vi "运维调试_总磷总氮.vi"() -> ()   [LabVIEW 2016, in "斯坦道氨氮.lvlib"]
uses:
  <vilib>/Utility/miscctls.llb/LVPointTypeDef.ctl
  <vilib>/Plasmionique/MB Master/MB_Master/MB_Master.lvclass
  <vilib>/Utility/config.llb/NI_LVConfig.lvlib
  <vilib>/ptbypt/NI_PtbyPt.lvlib
panel:
  out "权限等级":enum16{"一级权限", "二级权限", "三级权限", "超级权限"}(ring)
  out "试剂余量显示":sgl[][](graph)
  in  "仪器校准":bool
  in  "参数查询":bool
  out "简易步骤名称":string
  in  "温度曲线":bool
  in  "试剂余量":bool
  in  "灯值调整":bool
  in  "启动参数设置":bool
  out "固件版本号":string
  in  "定时设置":cluster{"启动":bool, "控制命令":T1, "测量参数":T2}(xcontrol)
  out "模块版本号":string
  out "注射器温度":sgl
  out "消解温度":sgl
  out "ADC":sgl
  out "F3":sgl format="%#.6f"
  out "F2":sgl format="%#.6f"
  out "F1":sgl format="%#.6f"
  out "F0":sgl format="%#.6f"
  out "运行状态":T3 {"数据时间:" format="%<%y/%m/%d %H:%M:%S>T"; "仪器时间:" format="%<%y/%m/%d %H:%M:%S>T"}
  in  "单选按钮":T4(radio)=enum."总氮"
  out "布尔":bool
  in  "流程固件":bool
  out "字符串 2":string
  in  "数组":string[](array[string])
  in  "返回":bool
  in  "参数设置":bool
  out "集成报警信息":string
  in  "停止":bool
  in  "手动启动":bool
  in  "调试":bool
  out "多列列表框":i32(listbox)
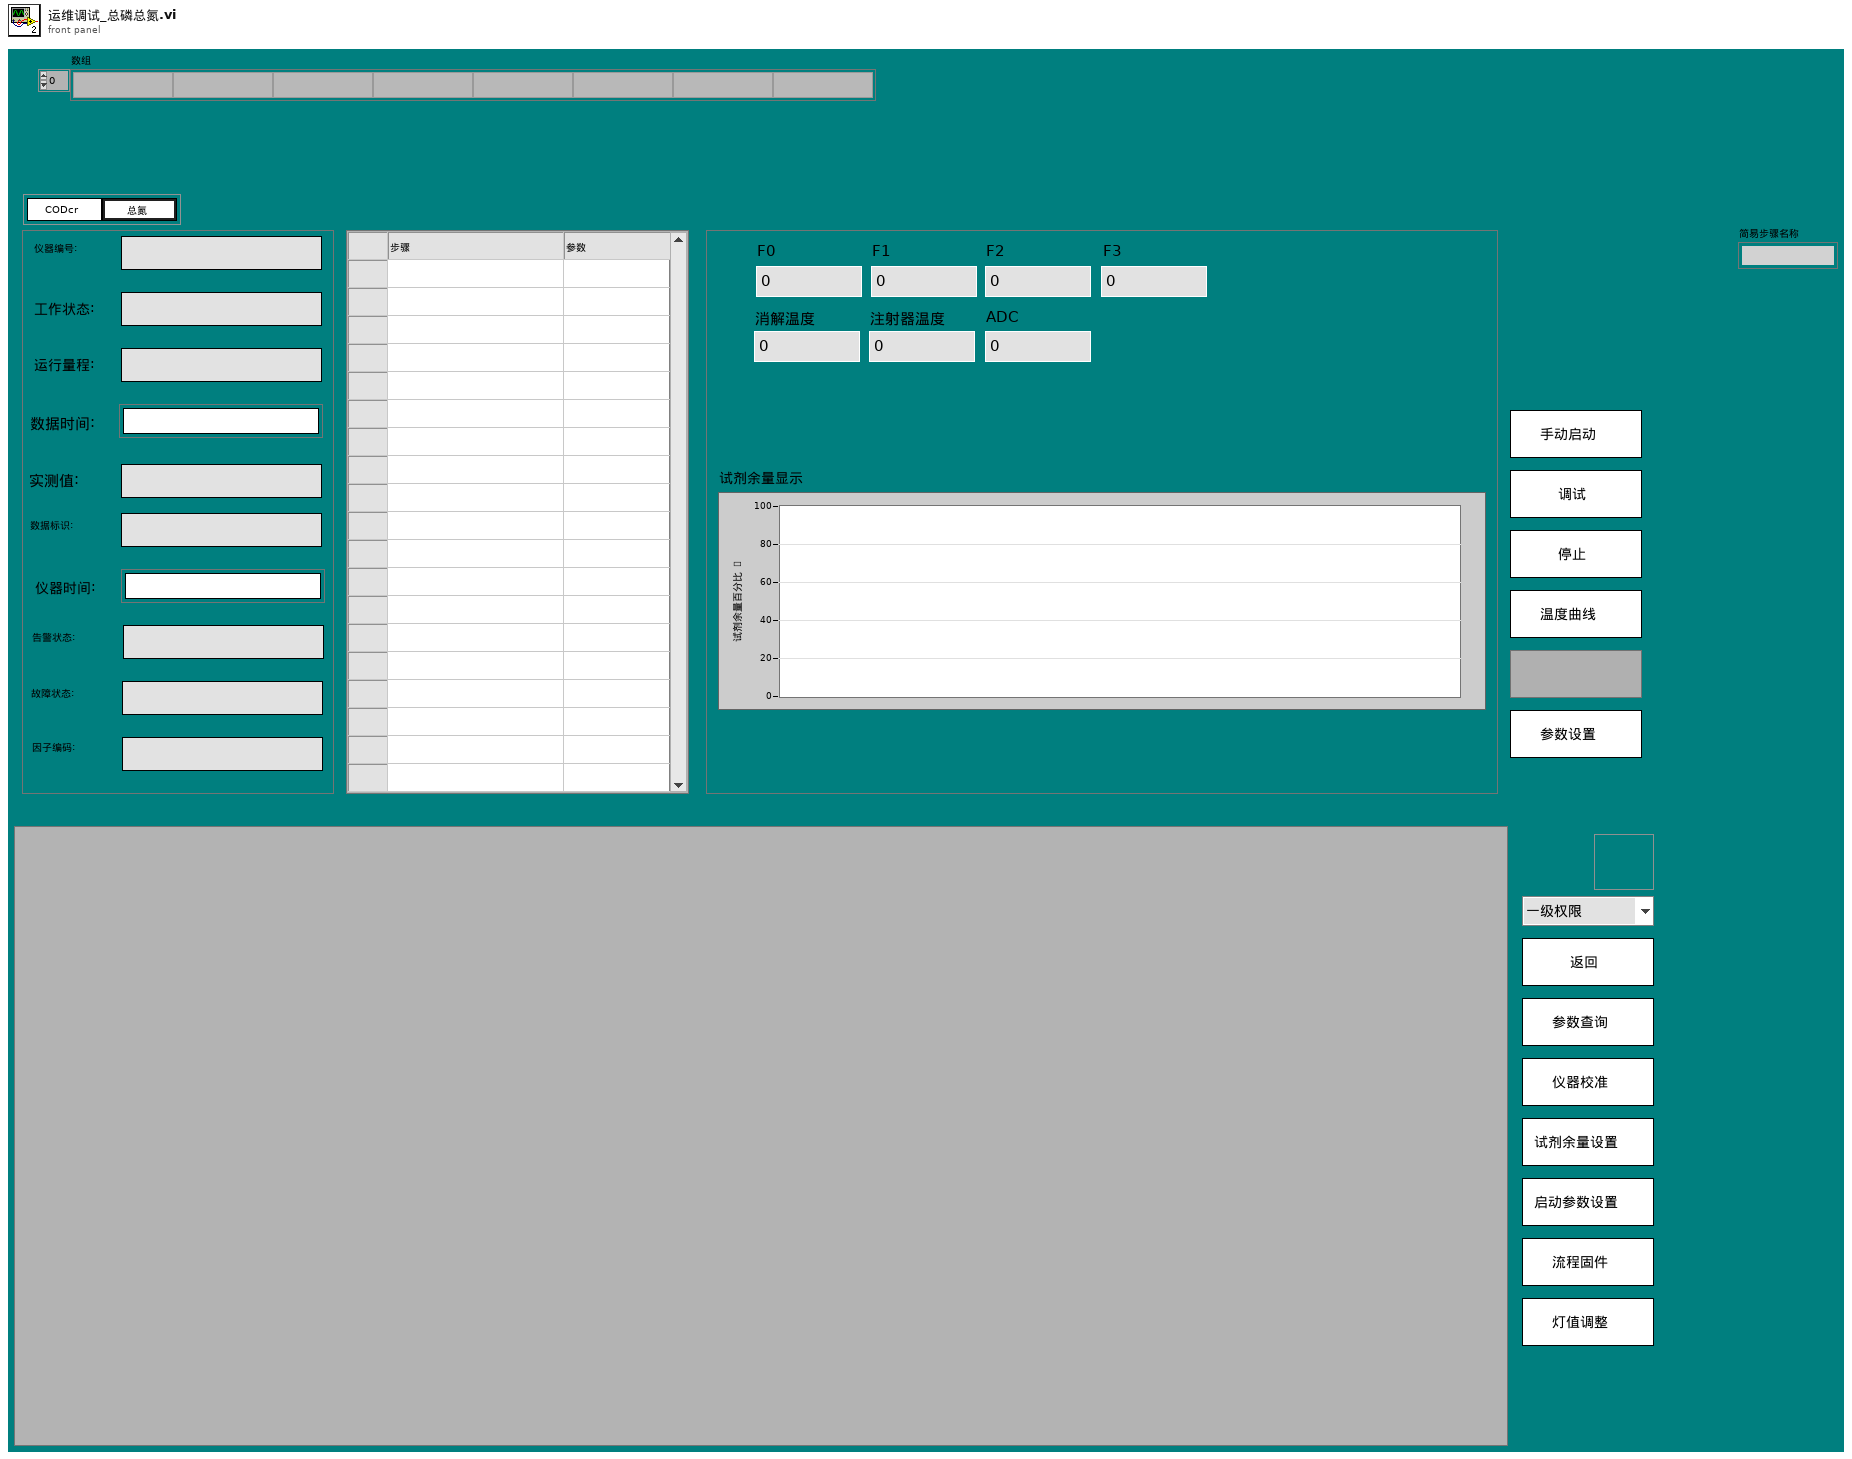
[diagram p1: front panel]
types:
  T1 = typedef "定时设置.xctl/国标控制命令.ctl" = enum16{"启动测量", "标样核查", "零点核查", "跨度核查", "空白测试", "平行样测试", "加标回收", "空白校准", "标样校准", "初始化（清洗）", "停止测试", "仪器重启", "校时", "模式设置", "测量间隔设置"}
  T2 = typedef "定时设置.xctl/测量参数.ctl" = u16
  T3 = cluster{"仪器编号:":string, "工作状态:":string, "运行量程: ":string, "数据时间:":timestamp, "实测值:":string, "数据标识: ":string, "仪器时间:":timestamp, "告警状态: ":string, "故障状态:  ":string, "因子编码:":string}
  T4 = enum32{"COD", "氨氮", "总氮", "总磷", "磷酸盐", "硝氮", "亚硝氮", "硅酸盐", "硫化物"}
  T5 = cluster{"时间源选择":enum16{"系统时间源", "仪器时间源"}, "外部时间源":timestamp}
  T6 = cluster{"系统时间":timestamp, "工作状态":u16, "测量模式":enum16{"待机", "连续模式", "周期模式", "定点模式", "受控模式", "手动模式"}, "告警代码":u16, "故障代码":u16, "日志代码":u16, "软件版本":u16, "F0":sgl, "F1":sgl, "F2":sgl, "F3":sgl, "T":sgl, "H":sgl, "id":u16, "flowid":u16, "量程":u16, "总磷控温温度1":sgl, "营养盐控温温度2":sgl, "ADC":sgl}
  T7 = enum32{"Bad", "Idle", "Run top level", "Running"}
  T8 = cluster{"Major":u16, "Minor":u16, "Fix":u16, "Build":u16}
  T9 = typedef "LVPointTypeDef.ctl" = cluster{"Horizontal":i16, "Vertical":i16}
  T10 = cluster{"因子编码":u32, "单位":u16, "标样参考值":sgl, "水样数据时间":timestamp, "水样实测值":sgl, "水样数据标识":string, "标样数据时间":timestamp, "标样实测值":sgl, "标样数据标识":string, "空白数据时间":timestamp, "空白实测值":sgl, "空白数据标识":string, "零点核查数据时间":timestamp, "零点核查实测值":sgl, "零点核查数据标识":string, "跨度核查数据时间":timestamp, "跨度核查实测值":sgl, "跨度核查数据标识":string, "加标回收数据时间":timestamp, "加标回收实测值":sgl, "加标回收数据标识":string, "平行样数据时间":timestamp, "平行样实测值":sgl, "平行样数据标识":string, "F0":sgl, "F1":sgl, "F2":sgl, "F3":sgl, "F4":sgl, "F5":sgl, "F6":sgl, "F7":sgl, "温度":sgl, "湿度":sgl, "X值":sgl, "fidrange":u16}[]
  T11 = cluster{"因子编码":u32, "单位":u16, "标样参考值":sgl, "水样数据时间":timestamp, "水样实测值":sgl, "水样数据标识":string, "标样数据时间":timestamp, "标样实测值":sgl, "标样数据标识":string, "空白数据时间":timestamp, "空白实测值":sgl, "空白数据标识":string, "零点核查数据时间":timestamp, "零点核查实测值":sgl, "零点核查数据标识":string, "跨度核查数据时间":timestamp, "跨度核查实测值":sgl, "跨度核查数据标识":string, "加标回收数据时间":timestamp, "加标回收实测值":sgl, "加标回收数据标识":string, "平行样数据时间":timestamp, "平行样实测值":sgl, "平行样数据标识":string, "F0":sgl, "F1":sgl, "F2":sgl, "F3":sgl, "F4":sgl, "F5":sgl, "F6":sgl, "F7":sgl, "温度":sgl, "湿度":sgl, "X值":sgl, "fidrange":u16}
  T12 = cluster{"时间标识":timestamp, "设备":string, "日志信息":string, "备注":string}
  T13 = cluster{"参数":string, "报警内容":string, "报警分析":string}
  T14 = typedef "NI_LVConfig.lvlib/Config Data RefNum.ctl" = refnum<k1>
  T15 = cluster{"时间标识":timestamp, "设备":string, "日志信息":string, "流程参数":string}
  T16 = typedef "LVRowAndColumnUnsignedTypeDef.ctl" = cluster{"Row":u32, "Column":u32}
  T17 = enum16{"空闲", "水样测试", "标样核查", "零点核查", "跨度核查", "空白测试", "平行样测试", "加标回收", "空白校准", "标样校准", "初始化（清洗）"}
  T18 = cluster{"站号":u16, "量程切换":enum32{"H", "L", "AUTO"}, "控制命令":enum16{"启动测量", "标样核查", "零点核查", "跨度核查", "空白测试", "平行样测试", "加标回收", "空白校准", "标样校准", "初始化（清洗）", "停止测试", "仪器重启", "校时", "模式设置", "测量间隔设置"}, "模式设置":enum16{"待机", "连续模式", "周期模式", "定点模式", "受控模式", "手动模式"}, "测量间隔":u16}
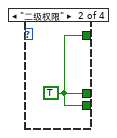
[diagram p9: hidden frame]
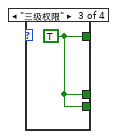
[diagram p10: hidden frame]
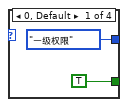
[diagram p11: hidden frame]
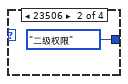
[diagram p12: hidden frame]
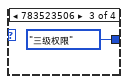
[diagram p13: hidden frame]
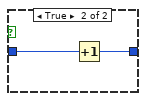
[diagram p15: hidden frame]
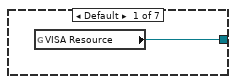
[diagram p17: hidden frame]
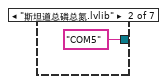
[diagram p18: hidden frame]
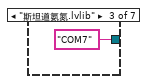
[diagram p19: hidden frame]
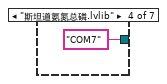
[diagram p20: hidden frame]
diagram:
  n1 = while {
    stop <- FALSE stop-if-true
    n2 = vi-ref "测量流程.vi"() -> (w39:refnum<vi>)
    n3 = global read "VAR总磷总氮全局变量.vi" "状态告警区"() -> (w36:T6)
    n4 = Wait (ms)(milliseconds to wait=u32 500 ("等待时间（毫秒）")) -> ()  [unwired: 1 out]
    n5 = Unbundle By Name("定时设置") -> ("启动"=w33:bool, "控制命令"=w32:T1)
    n6 = property class="VI"(reference=w39) -> ("Exec.State"=w38:T7, "Name"=w37:string)  [unwired: 1 in, 2 out]
    n7 = Unbundle By Name(w36) -> ("工作状态"=w35:u16, "系统时间"=w30:timestamp)
    n8 = case shown="真" w33 {
      tunnel: w37 -> [_ w46]
      tunnel: w32 -> [_ w45]
      tunnel: w38 -> [_ w44]
      frame False {
      }
      frame True {
        n9 = case shown="\"Idle\"" w44 {
          tunnel: w46 -> [_ w50]
          tunnel: w45 -> [_ w47]
          frame "Bad", Default {
          }
          frame "Idle" {
            n10 = Open VI Reference(type specifier VI Refnum (for type only)=refnum<vi> refnum, vi path=w50, options=128 ("选项")) -> (vi reference=w51:refnum<vi>, error out=w52:errorcluster)  [unwired: 3 in]
            n11 = call-by-ref "开始异步调用"(reference=w51, error in=w52, "控制命令"=w47) -> (reference out=w53:refnum<vi>, error out=w54:errorcluster)  [unwired: 11 in]
            n12 = Close Reference(reference=w53, error in (no error)=w54) -> ()  [unwired: 1 out]
          }
        }
      }
    }
    n13 = case shown="0" w35 {
      tunnel: [FALSE TRUE] -> w28
      frame 0 {
      }
      frame 1, Default {
      }
    }
    n14 = Bundle By Name(cluster=T5 {"时间源选择"=enum."仪器时间源", "外部时间源"=timestamp(0 s since 1904-01-01)} ("时间源"), "外部时间源"=w30) -> (w29:T5)
    n15 = property on="定时设置" class="定时设置 (严格)"("仪器状态"=w28, "时间源"=w29) -> ()  [unwired: 2 in, 2 out]
  }
  n16 = flat-sequence {
    tunnel: [w56] -> w16
    tunnel: [w55] -> w14
    tunnel: w16 -> [w67]
    tunnel: [w67] -> w15
    tunnel: w14 -> [w72]
    tunnel: [w72] -> w13
    tunnel: w15 -> [w98]
    tunnel: [w98] -> w17
    tunnel: w13 -> [_]
    tunnel: w17 -> [w101]
    tunnel: [w164] -> w18
    frame #0 {
      n17 = control-ref of="本VI"() -> (w66:refnum<vi>)
      n18 = property class="VI"(reference=w66) -> ("Library.Version"=w65:T8)  [unwired: 1 in, 2 out]
      n19 = Unbundle By Name(w65) -> ("Major"=w63:u16, "Minor"=w62:u16, "Fix"=w61:u16, "Build"=w60:u16)
      n20 = control-ref of="本VI"() -> (w57:refnum<vi>)
      n21 = Format Into String(format string="模块版本号：%d.%d.%d.%d" ("格式字符串"), w63, w62, w61, w60) -> (resulting string=→"模块版本号":string)  [unwired: 2 in, 1 out]
      n22 = property class="VI"(reference=w57) -> ("Library"=w58:refnum<vi>)  [unwired: 1 in, 2 out]
      n23 = property class="Library"(reference=w58) -> ("LocalName"=w56:string)  [unwired: 1 in, 2 out]
      n24 = property on="定时设置" class="定时设置 (严格)"("引用参数"=w56) -> ()  [unwired: 2 in, 2 out]
      n25 = call "配置读取.vi"() -> ("error out"=w55:errorcluster)  [unwired: 11 in]
    }
    frame #1 {
      n26 = global read "总磷总氮断电保存全局变量.vi" "IP"() -> (w71:string)
      n27 = global read "总磷总氮断电保存全局变量.vi" "VISA Resource"() -> (w68:refnum<visa-resource-name>)
      n28 = Empty String/Path?(string/path=w71) -> (empty?=w70:bool)
      n29 = case shown="真" w70 {
        tunnel: w67 -> [_ w83]
        frame False {
        }
        frame True {
          n30 = case shown="\"斯坦道CODcr.lvlib\"" w83 {
            tunnel: [w84 "192.168.1.203" ("IP") "192.168.1.202" ("IP") "192.168.1.202" ("IP") "192.168.1.203" ("IP") "192.168.1.204" ("IP") "192.168.1.205" ("IP")] -> w82
            frame Default {
              n31 = global read "总磷总氮断电保存全局变量.vi" "IP"() -> (w84:string)
            }
            frame "斯坦道总磷总氮.lvlib" {
            }
            frame "斯坦道氨氮.lvlib" {
            }
            frame "斯坦道氨氮总磷.lvlib" {
            }
            frame "斯坦道总磷.lvlib" {
            }
            frame "斯坦道总氮.lvlib" {
            }
            frame "斯坦道CODcr.lvlib" {
            }
          }
          n32 = global write "总磷总氮断电保存全局变量.vi" "IP"(w82) -> ()
        }
      }
      n33 = Empty String/Path?(string/path=w68) -> (empty?=w69:bool)
      n34 = case shown="真" w69 {
        tunnel: w67 -> [_ w74]
        frame False {
        }
        frame True {
          n35 = case shown="\"斯坦道CODcr.lvlib\"" w74 {
            tunnel: [w75 "COM5" ("IP") "COM7" ("IP") "COM7" ("IP") "COM5" ("IP") "COM10" ("IP") "COM9" ("IP")] -> w73
            frame Default {
              n36 = global read "总磷总氮断电保存全局变量.vi" "VISA Resource"() -> (w75:refnum<visa-resource-name>)
            }
            frame "斯坦道总磷总氮.lvlib" {
            }
            frame "斯坦道氨氮.lvlib" {
            }
            frame "斯坦道氨氮总磷.lvlib" {
            }
            frame "斯坦道总磷.lvlib" {
            }
            frame "斯坦道总氮.lvlib" {
            }
            frame "斯坦道CODcr.lvlib" {
            }
          }
          n37 = global write "总磷总氮断电保存全局变量.vi" "VISA Resource"(w73) -> ()
        }
      }
    }
    frame #2 {
      n38 = global read "总磷总氮断电保存全局变量.vi" "MB通信方式选择"() -> (w94:enum16{"串口", "TCP"})
      n39 = global read "总磷总氮断电保存全局变量.vi" "VISA Resource"() -> (w93:refnum<visa-resource-name>)
      n40 = global read "总磷总氮断电保存全局变量.vi" "PORT"() -> (w96:string)
      n41 = Decimal String To Number(string=w96) -> (number=w95:i32)  [unwired: 2 in, 1 out]
      n42 = global read "总磷总氮断电保存全局变量.vi" "IP"() -> (w97:string)
      n43 = call "获取启动参数.vi"("MB通信方式选择"=w94, "Port (502)"=w95, "IP Address"=w97, "VISA Resource"=w93) -> ("error out"=w92:errorcluster, "数组"=w91:cluster{"String":string, "Value":u16}[])  [unwired: 6 in]
      n44 = case shown="无错误" w92 {
        tunnel: w91 -> [w99 _]
        frame No Error {
          n45 = flat-sequence {
            tunnel: w99 -> [w100]
            frame #0 {
              n46 = global write "总磷总氮断电保存全局变量.vi" "启动队列名称"(w100) -> ()
            }
            frame #1 {
              n47 = call "配置写入.vi"() -> ()  [unwired: 11 in, 1 out]
            }
          }
        }
        frame Error {
        }
      }
    }
    frame #3 {
      n48 = global read "总磷总氮断电保存全局变量.vi" "启动队列名称"() -> (w103:cluster{"String":string, "Value":u16}[])
      n49 = Empty Array?(array=w103) -> (empty?=w102:bool)
      n50 = case shown="真" w102 {
        tunnel: w101 -> [_ w104]
        frame False {
        }
        frame True {
          n51 = case shown="\"斯坦道CODcr.lvlib\"" w104 {
            frame Default {
            }
            frame "斯坦道总磷总氮.lvlib" {
              n52 = global write "总磷总氮断电保存全局变量.vi" "启动队列名称"(cluster{"String":string, "Value":u16}[] [{"String"="总氮", "Value"=2}, {"String"="总磷", "Value"=1}] ("启动队列名称")) -> ()
            }
            frame "斯坦道氨氮.lvlib" {
              n53 = global write "总磷总氮断电保存全局变量.vi" "启动队列名称"(cluster{"String":string, "Value":u16}[] [{"String"="氨氮", "Value"=3}] ("启动队列名称")) -> ()
            }
            frame "斯坦道氨氮总磷.lvlib" {
              n54 = global write "总磷总氮断电保存全局变量.vi" "启动队列名称"(cluster{"String":string, "Value":u16}[] [{"String"="氨氮", "Value"=3}, {"String"="总磷", "Value"=1}] ("启动队列名称")) -> ()
            }
            frame "斯坦道总磷.lvlib" {
              n55 = global write "总磷总氮断电保存全局变量.vi" "启动队列名称"(cluster{"String":string, "Value":u16}[] [{"String"="总磷", "Value"=1}] ("启动队列名称")) -> ()
            }
            frame "斯坦道总氮.lvlib" {
              n56 = global write "总磷总氮断电保存全局变量.vi" "启动队列名称"(cluster{"String":string, "Value":u16}[] [{"String"="总氮", "Value"=2}] ("启动队列名称")) -> ()
            }
            frame "斯坦道CODcr.lvlib" {
              n57 = global write "总磷总氮断电保存全局变量.vi" "启动队列名称"(cluster{"String":string, "Value":u16}[] [{"String"="CODcr", "Value"=22}] ("启动队列名称")) -> ()
            }
          }
        }
      }
    }
    frame #4 {
      # "初始化"
      n58 = global read "总磷总氮断电保存全局变量.vi" "流程路径"() -> (w112:path)
      n59 = global read "总磷总氮断电保存全局变量.vi" "启动队列名称"() -> (w117:cluster{"String":string, "Value":u16}[])
      n60 = global read "总磷总氮断电保存全局变量.vi" "启动队列名称"() -> (w115:cluster{"String":string, "Value":u16}[])
      n61 = call <vilib>:"Check if File or Folder Exists.vi"("path"=w112) -> ("file or folder exists?"=w111:bool)  [unwired: 8 in, 2 out]
      n62 = for {
        tunnel: w117 -> [w129] mode=indexing
        tunnel: [w128] -> w116 mode=indexing
        n63 = Unbundle By Name(w129) -> ("String"=w128:string)
      }
      n64 = for {
        tunnel: w115 -> [w127] mode=indexing
        shift-right: [w126] -> w114
        shift-left: "" -> [w124]
        n65 = Unbundle By Name(w127) -> ("String"=w125:string)
        n66 = Concatenate Strings(w124, w125) -> (w126:string)
      }
      n67 = property on="单选按钮" class="RadioBtnsControl (严格)"() -> ("Controls[]"=w118:refnum<vi>[])  [unwired: 2 in, 2 out]
      n68 = for {
        tunnel: w118 -> [w137] mode=indexing
        tunnel: w116 -> [w136]
        n69 = property class="Ctl"(reference=w137) -> (reference out=w135:refnum<vi>, "Label.Text"=w131:string)  [unwired: 1 in, 1 out]
        n70 = case shown="\"COD\"" w131 {
          selector: w131 -> [w138 _]
          tunnel: [w138 "CODcr"] -> w130
          frame Default {
          }
          frame "COD" {
          }
        }
        n71 = Search 1D Array(1D array=w136, element=w130) -> (index of element=w134:i32)  [unwired: 1 in]
        n72 = Not Equal?(x=w134, y=-1) -> (x != y?=w132:bool)
        n73 = property class="Ctl"(reference=w135, "Visible"=w132) -> ()  [unwired: 1 in, 2 out]
      }
      n74 = case shown="假" w111 {
        frame False {
          n75 = global read "总磷总氮断电保存全局变量.vi" "启动队列名称"() -> (w120:cluster{"String":string, "Value":u16}[])
          n76 = for {
            tunnel: w120 -> [w123] mode=indexing
            tunnel: [w122] -> w119 mode=indexing
            n77 = Unbundle By Name(w123) -> ("String"=w122:string)
          }
          n78 = call "获取默认流程路径.vi"("参数"=w119) -> ("路径"=w121:path)  [unwired: 10 in]
          n79 = global write "总磷总氮断电保存全局变量.vi" "流程路径"(w121) -> ()
        }
        frame True {
        }
      }
      n80 = global write "VAR总磷总氮全局变量.vi" "模块名称"(w114) -> ()
    }
    frame #5 {
      n81 = vi-ref "总磷总氮通讯.vi"() -> (w148:refnum<vi>)
      n82 = vi-ref "关键参数交互.vi"() -> (w147:refnum<vi>)
      n83 = vi-ref "总磷总氮测量数据储存.vi"() -> (w156:refnum<vi>)
      n84 = property class="VI"(reference=w148) -> ("Name"=w149:string)  [unwired: 1 in, 2 out]
      n85 = property class="VI"(reference=w156) -> ("Name"=w163:string)  [unwired: 1 in, 2 out]
      n86 = Open VI Reference(type specifier VI Refnum (for type only)=refnum<vi> refnum, vi path=w149, options=128 ("选项")) -> (vi reference=w151:refnum<vi>, error out=w153:errorcluster)  [unwired: 3 in]
      n87 = property class="VI"(reference=w147) -> ("Name"=w141:string)  [unwired: 1 in, 2 out]
      n88 = call-by-ref "开始异步调用"(reference=w151, error in=w153) -> (reference out=w155:refnum<vi>, error out=w154:errorcluster)  [unwired: 12 in]
      n89 = Open VI Reference(type specifier VI Refnum (for type only)=refnum<vi> refnum, vi path=w163, options=128 ("选项")) -> (vi reference=w161:refnum<vi>, error out=w159:errorcluster)  [unwired: 3 in]
      n90 = Close Reference(reference=w155, error in (no error)=w154) -> ()  [unwired: 1 out]
      n91 = Open VI Reference(type specifier VI Refnum (for type only)=refnum<vi> refnum, vi path=w141, options=128 ("选项")) -> (vi reference=w143:refnum<vi>, error out=w144:errorcluster)  [unwired: 3 in]
      n92 = call-by-ref "开始异步调用"(reference=w161, error in=w159) -> (reference out=w157:refnum<vi>, error out=w158:errorcluster)  [unwired: 12 in]
      n93 = call-by-ref "开始异步调用"(reference=w143, error in=w144) -> (reference out=w146:refnum<vi>, error out=w145:errorcluster)  [unwired: 12 in]
      n94 = Close Reference(reference=w157, error in (no error)=w158) -> ()  [unwired: 1 out]
      n95 = Close Reference(reference=w146, error in (no error)=w145) -> ()  [unwired: 1 out]
    }
    frame #6 {
      n96 = call "设置模块队列名.vi"() -> ("Msg"=w164:string)  [unwired: 5 in]
    }
  }
  n97 = call "配置文件路径.vi"() -> ("appended path"=w21:path)  [unwired: 11 in]
  n98 = call "时间延迟"() -> ("error out"=w27:errorcluster)  [unwired: 11 in]
  n99 = flat-sequence {
    frame #0 {
      n100 = property on="窗格" class="Pane"("Origin"=T9 {"Horizontal"=0, "Vertical"=0} ("原点")) -> ()  [unwired: 2 in, 2 out]
    }
  }
  n101 = while {
    shift-right: [w167] -> _
    shift-left: _ -> [w166]
    stop <- FALSE stop-if-true
    n102 = global read "VAR总磷总氮全局变量.vi" "状态告警区"() -> (w189:T6)
    n103 = global read "VAR总磷总氮全局变量.vi" "通讯状态"() -> (w201:bool)
    n104 = Wait (ms)(milliseconds to wait=u32 1000 ("等待时间（毫秒）")) -> ()  [unwired: 1 out]
    n105 = case shown="\"COD\", 默认" "单选按钮" {
      tunnel: [22 3 2 1 4 5 6 7 8] -> w168
      frame "COD", Default {
      }
      frame "氨氮" {
      }
      frame "总氮" {
      }
      frame "总磷" {
      }
      frame "磷酸盐" {
      }
      frame "硝氮" {
      }
      frame "亚硝氮" {
      }
      frame "硅酸盐" {
      }
      frame "硫化物" {
      }
    }
    n106 = Unbundle By Name(w189) -> ("id"=w188:u16, "工作状态"=w183:u16)
    n107 = case shown="真" w201 {
      tunnel: ["通讯异常" ("集成报警信息") w295] -> w200
      frame False {
      }
      frame True {
        n108 = global read "VAR总磷总氮全局变量.vi" "状态告警区"() -> (w301:T6)
        n109 = Unbundle By Name(w301) -> ("工作状态"=w300:u16)
        n110 = feedback #1(0) -> (w298:i32)
        n111 = case shown="默认" w300 {
          tunnel: w298 -> [_ w303]
          tunnel: [_ w302] -> w296
          frame 0 {
          }
          frame Default {
            n112 = Increment(x=w303) -> (x+1=w302:i32)
          }
        }
        n113 = feedback-in #1(w296) -> ()
        n114 = global read "VAR总磷总氮全局变量.vi" "测量状态"() -> (w294:string)
        n115 = Format Into String(format string="工作计时: %d 秒" ("格式字符串"), initial string=w294, w296) -> (resulting string=w295:string)  [unwired: 1 in, 1 out]
      }
    }
    "集成报警信息" <- w200
    n116 = global read "VAR总磷总氮全局变量.vi" "测量数据区数组"() -> (w172:T10)
    n117 = case shown="1, 默认" w183 {
      tunnel: w188 -> [_ w246]
      frame 0 {
      }
      frame 1, Default {
        n118 = case shown="8" w246 {
          frame 0, Default {
          }
          frame 1 {
            n119 = local write "单选按钮"(T4."总磷" ("单选按钮")) -> ()
          }
          frame 2 {
            n120 = local write "单选按钮"(T4."总氮" ("单选按钮")) -> ()
          }
          frame 22 {
            n121 = local write "单选按钮"(T4."COD" ("单选按钮")) -> ()
          }
          frame 3 {
            n122 = local write "单选按钮"(T4."氨氮" ("单选按钮")) -> ()
          }
          frame 4 {
            n123 = local write "单选按钮"(T4."磷酸盐" ("单选按钮")) -> ()
          }
          frame 5 {
            n124 = local write "单选按钮"(T4."硝氮" ("单选按钮")) -> ()
          }
          frame 6 {
            n125 = local write "单选按钮"(T4."亚硝氮" ("单选按钮")) -> ()
          }
          frame 7 {
            n126 = local write "单选按钮"(T4."硅酸盐" ("单选按钮")) -> ()
          }
          frame 8 {
            n127 = local write "单选按钮"(T4."硫化物" ("单选按钮")) -> ()
          }
        }
      }
    }
    n128 = global read "VAR总磷总氮全局变量.vi" "状态告警区"() -> (w199:T6)
    n129 = call "id参数转换.vi"("id"=w168) -> ("数组资源索引"=w169:i32)  [unwired: 9 in, 1 out]
    n130 = Unbundle By Name(w199) -> ("系统时间"=w195:timestamp, "工作状态"=w194:u16, "告警代码"=w187:u16, "故障代码"=w185:u16, "量程"=w192:u16)
    n131 = Index Array(array=w172, index=w169) -> (element=w171:T11)
    n132 = case shown="8" w194 {
      selector: w194 -> [w260 _ w266 w268 w270 w272 w274 w276 w278 w280 w282 w284 w286 w288]
      tunnel: [w261 "空闲" ("工作状态") "水样测量" ("工作状态") "标样核查" ("工作状态") "零点核查" ("工作状态") "跨度核查" ("工作状态") "空白测试" ("工作状态") "平行样测试" ("工作状态") "加标回收" ("工作状态") "空白校准" ("工作状态") "标样校准" ("工作状态") "初始化" ("工作状态") "单步调试" ("工作状态") w290] -> w193
      tunnel: [w259 w264 w266 w268 w270 w272 w274 w276 w278 w280 w282 w284 w286 w288] -> w167
      tunnel: w166 -> [w259 w264 _ _ _ _ _ _ _ _ _ _ _ _]
      frame Default {
        n133 = Format Into String(format string="%d" ("格式字符串"), initial string="未知" ("工作状态"), w260) -> (resulting string=w261:string)  [unwired: 1 in, 1 out]
      }
      frame 0 {
      }
      frame 1 {
      }
      frame 2 {
      }
      frame 3 {
      }
      frame 4 {
      }
      frame 5 {
      }
      frame 6 {
      }
      frame 7 {
      }
      frame 8 {
      }
      frame 9 {
      }
      frame 10 {
      }
      frame 254 {
      }
      frame 255 {
        n134 = local read "简易步骤名称"() -> (w291:string)
        n135 = Format Into String(format string="(%s)" ("格式字符串"), initial string="简易流程" ("工作状态"), w291) -> (resulting string=w290:string)  [unwired: 1 in, 1 out]
      }
    }
    n136 = case shown="5, 8" w166 {
      tunnel: [w215 w221 w225 w229 w233 w237 w241 w245] -> w182
      tunnel: [w213 w220 w224 w228 w231 w236 w240 w244] -> w177
      tunnel: [w216 w219 w223 w227 w230 w235 w239 w243] -> w175
      tunnel: w171 -> [_ w218 w222 w226 w232 w234 w238 w242]
      frame 0, Default {
        n137 = local read "运行状态"() -> (w217:T3)
        n138 = Unbundle By Name(w217) -> ("数据时间:"=w215:timestamp, "实测值:"=w214:string, "数据标识:"=w216:string)
        n139 = Fract/Exp String To Number(string=w214) -> (number=w213:dbl)  [unwired: 3 in, 1 out]
      }
      frame 1 {
        n140 = Unbundle By Name(w218) -> ("水样数据时间"=w221:timestamp, "水样实测值"=w220:sgl, "水样数据标识"=w219:string)
      }
      frame 2, 9 {
        n141 = Unbundle By Name(w222) -> ("标样数据时间"=w225:timestamp, "标样实测值"=w224:sgl, "标样数据标识"=w223:string)
      }
      frame 3 {
        n142 = Unbundle By Name(w226) -> ("零点核查数据时间"=w229:timestamp, "零点核查实测值"=w228:sgl, "零点核查数据标识"=w227:string)
      }
      frame 4 {
        n143 = Unbundle By Name(w232) -> ("跨度核查数据时间"=w233:timestamp, "跨度核查实测值"=w231:sgl, "跨度核查数据标识"=w230:string)
      }
      frame 7 {
        n144 = Unbundle By Name(w234) -> ("加标回收数据时间"=w237:timestamp, "加标回收实测值"=w236:sgl, "加标回收数据标识"=w235:string)
      }
      frame 5, 8 {
        n145 = Unbundle By Name(w238) -> ("空白数据时间"=w241:timestamp, "空白实测值"=w240:sgl, "空白数据标识"=w239:string)
      }
      frame 6 {
        n146 = Unbundle By Name(w242) -> ("平行样数据时间"=w245:timestamp, "平行样实测值"=w244:sgl, "平行样数据标识"=w243:string)
      }
    }
    n147 = Unbundle By Name(w171) -> ("因子编码"=w173:u32)
    n148 = global write "VAR总磷总氮全局变量.vi" "最近一次工作状态"(w166) -> ()
    n149 = case shown="1" w192 {
      tunnel: ["" ("字符串") "低量程 " ("字符串") "高量程 " ("字符串")] -> w191
      frame Default {
      }
      frame 0 {
      }
      frame 1 {
      }
    }
    n150 = Number To Fractional String(number=w177, precision (6)=i16 4 ("精度(6)")) -> (F-format string=w179:string)  [unwired: 2 in]
    n151 = global read "VAR总磷总氮全局变量.vi" "序列号"() -> (w196:string)
    n152 = Concatenate Strings(w179, " " ("字符串"), "mg/L" ("字符串")) -> (w176:string)
    n153 = Format Into String(format string="w%05d" ("格式字符串"), w173) -> (resulting string=w190:string)  [unwired: 2 in, 1 out]
    n154 = call "告警码字段定义.vi"("告警代码"=w187) -> ("字符串"=w186:string)  [unwired: 8 in, 2 out]
    n155 = call "故障码字段定义.vi"("故障代码"=w185) -> ("字符串"=w184:string)  [unwired: 10 in]
    n156 = Bundle By Name(cluster=T3 {"仪器编号:"="", "工作状态:"="", "运行量程: "="", "数据时间:"=timestamp(0 s since 1904-01-01), "实测值:"="", "数据标识: "="", "仪器时间:"=timestamp(0 s since 1904-01-01), "告警状态: "="", "故障状态:  "="", "因子编码:"=""} ("运行状态"), "仪器编号:"=w196, "仪器时间:"=w195, "工作状态:"=w193, "告警状态:"=w186, "故障状态:"=w184, "运行量程:"=w191, "数据时间:"=w182, "实测值:"=w176, "数据标识:"=w175, "因子编码:"=w190) -> (→"运行状态":T3)
  }
  n157 = call "Create balloon 队列.vi"() -> ("队列输出"=w24:refnum<queue>)  [unwired: 11 in]
  n158 = while {
    shift-right: [w307] -> _
    shift-left: _ -> [w306]
    stop <- FALSE stop-if-true
    n159 = global read "VAR总磷总氮全局变量.vi" "状态告警区"() -> (w309:T6)
    n160 = Wait (ms)(milliseconds to wait=u32 1000 ("等待时间（毫秒）")) -> ()  [unwired: 1 out]
    n161 = Unbundle By Name(w309) -> ("工作状态"=w308:u16, "总磷控温温度1"=w305:sgl, "营养盐控温温度2"=w304:sgl)
    n162 = case shown="默认" w308 {
      tunnel: [TRUE _] -> w307
      tunnel: w306 -> [w318 _]
      tunnel: w305 -> [w316 _]
      tunnel: w304 -> [w314 _]
      frame Default {
        n163 = case shown="真" w318 {
          tunnel: [_ w321] -> w317
          tunnel: [_ w320] -> w315
          frame False {
          }
          frame True {
            n164 = global read "VAR总磷总氮全局变量.vi" "波形图-消解温度"() -> (w321:dbl[])
            n165 = global read "VAR总磷总氮全局变量.vi" "波形图-注射器温度"() -> (w320:dbl[])
          }
        }
        n166 = Insert Into Array(array=w317, new element=w316) -> (w313:dbl[])  [unwired: 1 in]
        n167 = Insert Into Array(array=w315, new element=w314) -> (w312:dbl[])  [unwired: 1 in]
        n168 = global write "VAR总磷总氮全局变量.vi" "波形图-消解温度"(w313) -> ()
        n169 = global write "VAR总磷总氮全局变量.vi" "波形图-注射器温度"(w312) -> ()
      }
      frame 0, 254, 255 {
      }
    }
  }
  n170 = while {
    shift-right: [w333] -> _
    shift-left: u32 0 ("y") -> [w335]
    stop <- FALSE stop-if-true
    # "密码权限"
    n171 = local read "布尔"() -> (w336:bool)
    n172 = Wait (ms)(milliseconds to wait=u32 1000 ("等待时间（毫秒）")) -> ()  [unwired: 1 out]
    n173 = case shown="假" w336 {
      tunnel: w335 -> [_ w348]
      tunnel: [_ w347] -> w333
      frame False {
      }
      frame True {
        n174 = Increment(x=w348) -> (x+1=w347:u32)
      }
    }
    n175 = global read "VAR总磷总氮全局变量.vi" "权限等级"() -> (→"权限等级":enum16{"一级权限", "二级权限", "三级权限", "超级权限"})
    n176 = Greater Or Equal?(x=w333, y=u32 300) -> (x >= y?=w331:bool)
    n177 = case shown="真" w331 {
      frame False {
      }
      frame True {
        n178 = global write "VAR总磷总氮全局变量.vi" "权限密码"(u32 0 ("权限密码")) -> ()
      }
    }
    n179 = global read "VAR总磷总氮全局变量.vi" "权限密码"() -> (w328:u32)
    n180 = global read "VAR总磷总氮全局变量.vi" "权限等级"() -> (w325:enum16{"一级权限", "二级权限", "三级权限", "超级权限"})
    n181 = case shown="783523103" w328 {
      tunnel: [enum16{"一级权限", "二级权限", "三级权限", "超级权限"}."一级权限" ("权限等级") enum16{"一级权限", "二级权限", "三级权限", "超级权限"}."二级权限" ("权限等级") enum16{"一级权限", "二级权限", "三级权限", "超级权限"}."三级权限" ("权限等级") enum16{"一级权限", "二级权限", "三级权限", "超级权限"}."超级权限" ("权限等级")] -> w329
      tunnel: [TRUE _ _ _] -> w327
      frame 0, Default {
      }
      frame 23506 {
      }
      frame 783523506 {
      }
      frame 783523103 {
      }
    }
    n182 = case shown="\"超级权限\"" w325 {
      tunnel: [_ w338 w339 w340] -> w324
      tunnel: [_ w338 w339 w340] -> w323
      tunnel: [_ w338 w339 w340] -> w322
      frame "一级权限", Default {
      }
      frame "二级权限" {
        w338 = TRUE
      }
      frame "三级权限" {
        w339 = TRUE
      }
      frame "超级权限" {
        w340 = TRUE
      }
    }
    n183 = property on="灯值调整" class="Bool"("Visible"=w324) -> ()  [unwired: 2 in, 2 out]
    n184 = property on="流程固件" class="Bool"("Visible"=w322) -> ()  [unwired: 2 in, 2 out]
    n185 = property on="启动参数设置" class="Bool"("Visible"=w323) -> ()  [unwired: 2 in, 2 out]
    n186 = global write "VAR总磷总氮全局变量.vi" "权限等级"(w329) -> ()
    n187 = Not(x=w327) -> (.not. x?=→"布尔":bool)
  }
  n188 = while {
    tunnel: w24 -> [w355]
    shift-right: [w351] -> _
    shift-left: _ -> [w352]
    stop <- FALSE stop-if-true
    n189 = global read "VAR总磷总氮全局变量.vi" "状态告警区"() -> (w349:T6)
    n190 = Wait (ms)(milliseconds to wait=u32 100) -> ()  [unwired: 1 out]
    n191 = Unbundle By Name(w349) -> ("工作状态"=w350:u16, "id"=w357:u16, "日志代码"=w356:u16, "故障代码"=w354:u16, "告警代码"=w353:u16)
    n192 = case shown="1, 默认" w350 {
      tunnel: w357 -> [_ w372]
      tunnel: w356 -> [_ w371]
      tunnel: w355 -> [_ w368]
      tunnel: w354 -> [_ w367]
      tunnel: w353 -> [_ w366]
      tunnel: w352 -> [w360 w365]
      tunnel: [w360 w364] -> w351
      frame 0 {
      }
      frame 1, Default {
        n193 = call "id参数转换.vi"("id"=w372) -> ("table输出"=w369:string)  [unwired: 9 in, 1 out]
        n194 = Add(x=w367, y=w366) -> (x+y=w364:u16)
        n195 = Not Equal?(x=w364, y=w365) -> (x != y?=w362:bool)
        n196 = Not Equal To 0?(x=w364) -> (x != 0?=w363:bool)
        n197 = call "故障告警分析.vi"("告警代码"=w366, "故障代码"=w367, "运行步序"=w371, "参数"=w369) -> ("报警内容"=w370:T13)  [unwired: 6 in, 1 out]
        n198 = And(x=w363, y=w362) -> (x .and. y?=w361:bool)
        n199 = case shown="真" w361 {
          tunnel: w370 -> [_ w381]
          tunnel: w368 -> [_ w380]
          frame False {
          }
          frame True {
            n200 = Unbundle By Name(w381) -> ("参数"=w376:string, "报警内容"=w375:string, "报警分析"=w374:string)
            n201 = Get Date/Time In Seconds() -> (seconds since 1Jan1904=w379:timestamp)
            n202 = Bundle("报警内容"=w375, "报警分析"=w374) -> (w373:cluster{"报警内容":string, "报警分析":string})  [unwired: 1 in]
            n203 = Bundle By Name(cluster=T12 {"时间标识"=timestamp(0 s since 1904-01-01), "设备"="", "日志信息"="", "备注"=""} ("data in"), "时间标识"=w379, "设备"=w376, "日志信息"=w375, "备注"=w374) -> (w378:T12)
            n204 = call "balloon入队列.vi"("报警内容"=w373, "队列"=w380) -> ()  [unwired: 9 in, 1 out]
            n205 = call "总磷总氮报警信息.vi"("data in"=w378) -> ()  [unwired: 10 in, 1 out]
          }
        }
      }
    }
  }
  n206 = Read from Text File(file (use dialog)=w21) -> (text=w22:string)  [unwired: 3 in, 3 out]
  n207 = while {
    shift-right: [w384] -> _
    shift-left: w22 -> [w386]
    tunnel: w21 -> [w383]
    stop <- FALSE stop-if-true
    n208 = Read from Text File(file (use dialog)=w383) -> (text=w384:string)  [unwired: 3 in, 3 out]
    n209 = Not Equal?(x=w386, y=w384) -> (x != y?=w385:bool)
    n210 = Wait (ms)(milliseconds to wait=u32 1000 ("等待时间（毫秒）")) -> ()  [unwired: 1 out]
    n211 = case shown="真" w385 {
      tunnel: w383 -> [_ w388]
      frame False {
      }
      frame True {
        n212 = vi-ref "总磷总氮断电保存全局变量.vi"() -> (w392:refnum<vi>)
        n213 = call <vilib>:"Open Config Data.vi"("configuration file path"=w388) -> ("error out"=w390:errorcluster, "refnum"=w393:T14)  [unwired: 8 in, 1 out]
        n214 = call <userlib>:"Read Panel from INI__ogtk.vi"("error in (no error)"=w390, "VI ref"=w392, "refnum"=w393) -> ("error out"=w389:errorcluster, "refnum out"=w391:T14)  [unwired: 7 in]
        n215 = call <vilib>:"Close Config Data.vi"("error in (no error)"=w389, "refnum"=w391) -> ()  [unwired: 8 in, 2 out]
      }
    }
  }
  n216 = while {
    tunnel: w27 -> [_]
    stop <- FALSE stop-if-true
    n217 = global read "VAR总磷总氮全局变量.vi" "状态告警区"() -> (w422:T6)
    n218 = global read "VAR总磷总氮全局变量.vi" "状态告警区"() -> (w421:T6)
    n219 = global read "VAR总磷总氮全局变量.vi" "状态告警区"() -> (w419:T6)
    n220 = global read "VAR总磷总氮全局变量.vi" "状态告警区"() -> (w423:T6)
    n221 = Wait (ms)(milliseconds to wait=u32 1000 ("等待时间（毫秒）")) -> ()  [unwired: 1 out]
    n222 = Unbundle By Name(w423) -> ("id"=w397:u16, "flowid"=w396:u16, "量程"=w395:u16, "工作状态"=w399:u16, "日志代码"=w394:u16, "F0"=→"F0":sgl, "F1"=→"F1":sgl, "F2"=→"F2":sgl, "F3"=→"F3":sgl, "ADC"=→"ADC":sgl, "总磷控温温度1"=→"消解温度":sgl, "营养盐控温温度2"=→"注射器温度":sgl)
    n223 = Unbundle By Name(w419) -> ("日志代码"=w418:u16)
    n224 = Unbundle By Name(w422) -> ("日志代码"=w415:u16)
    n225 = Unbundle By Name(w421) -> ("工作状态"=w410:u16, "id"=w411:u16)
    n226 = case shown="0" w410 {
      frame 0 {
        n227 = local write "数组"(string[] [] ("数组")) -> ()
      }
      frame 1, Default {
      }
    }
    n228 = feedback-in #2(w415) -> ()
    n229 = feedback #2(w415) -> (w425:u16)
    n230 = feedback #3(w418) -> (w420:u16)
    n231 = feedback-in #3(w418) -> ()
    n232 = Not Equal To 0?(x=w410) -> (x != 0?=w408:bool)
    n233 = Subtract(x=w415, y=1) -> (x-y=→"多列列表框":i32)
    n234 = Not Equal?(x=w415, y=w425) -> (x != y?=w424:bool)
    n235 = Not Equal?(x=w418, y=w420) -> (x != y?=w417:bool)
    n236 = call <vilib>:"Boolean Crossing PtByPt.vi"("direction"=enum16{"either", "false-true", "true-false"}."false-true", "input"=w408) -> ("crossing"=w412:bool)  [unwired: 1 in]
    n237 = call <vilib>:"Boolean Crossing PtByPt.vi"("direction"=enum16{"either", "false-true", "true-false"}."true-false", "input"=w408) -> ("crossing"=w407:bool)  [unwired: 1 in]
    n238 = Bundle("id"=w397, "flowid"=w396, "量程"=w395) -> (w398:cluster{"id":u16, "flowid":u16, "量程":u16})  [unwired: 1 in]
    n239 = case shown="真" w424 {
      tunnel: w415 -> [_ w592]
      frame False {
      }
      frame True {
        n240 = Subtract(x=w592, y=1) -> (x-y=w590:i32)
        n241 = Subtract(x=w590, y=5) -> (x-y=w594:i32)
        n242 = Greater Or Equal To 0?(x=w594) -> (x >= 0?=w593:bool)
        n243 = property on="多列列表框" class="MCListbox (严格)"() -> (error out=w598:errorcluster, "TopLeft"=w599:T16)  [unwired: 2 in, 1 out]
        n244 = Select(t=w594, s=w593, f=0) -> (s? t:f=w595:i32)
        n245 = Bundle By Name(cluster=w599, "Row"=w595) -> (w600:T16)
        n246 = property on="多列列表框" class="MCListbox (严格)"(error in=w598, "TopLeft"=w600) -> ()  [unwired: 1 in, 2 out]
      }
    }
    n247 = case shown="真" w412 {
      tunnel: w410 -> [_ w465]
      tunnel: w411 -> [_ w462]
      frame False {
      }
      frame True {
        n248 = case shown="8" w465 {
          selector: w465 -> [w472 _ _ _ _ _ _ _ _ _ _ _]
          tunnel: [w471 "【水样测试】" ("字符串") "【标样核查】" ("字符串") "【零点核查】" ("字符串") "【跨度核查】" ("字符串") "【空白测试】" ("字符串") "【平行样测试】" ("字符串") "【加标回收】" ("字符串") "【空白校准】" ("字符串") "【标样校准】" ("字符串") "【单步调试】" ("字符串") "【简易步骤】" ("字符串")] -> w470
          frame 0, Default {
            n249 = Number To Decimal String(number=w472) -> (decimal integer string=w471:string)  [unwired: 1 in]
          }
          frame 1 {
          }
          frame 2 {
          }
          frame 3 {
          }
          frame 4 {
          }
          frame 5 {
          }
          frame 6 {
          }
          frame 7 {
          }
          frame 8 {
          }
          frame 9 {
          }
          frame 254 {
          }
          frame 255 {
          }
        }
        n250 = Concatenate Strings("<<" ("字符串"), w470, "启动" ("字符串")) -> (w469:string)
        n251 = call "id参数转换.vi"("id"=w462) -> ("table输出"=w461:string)  [unwired: 9 in, 1 out]
        n252 = Get Date/Time In Seconds() -> (seconds since 1Jan1904=w467:timestamp)
        n253 = Bundle By Name(cluster=T15 {"时间标识"=timestamp(0 s since 1904-01-01), "设备"="", "日志信息"="", "流程参数"=""} ("data in"), "时间标识"=w467, "设备"=w461, "日志信息"=w469) -> (w466:T15)
        n254 = call "总磷总氮操作日志.vi"("data in"=w466) -> ()  [unwired: 11 in]
      }
    }
    n255 = case shown="真" w407 {
      tunnel: w410 -> [_ w429]
      tunnel: w411 -> [_ w442]
      frame False {
      }
      frame True {
        n256 = case shown="6" w429 {
          selector: w429 -> [w449 _ _ _ _ _ _ _ _ _ _ _]
          tunnel: [w448 "【水样测试】" ("字符串") "【标样核查】" ("字符串") "【零点核查】" ("字符串") "【跨度核查】" ("字符串") "【空白测试】" ("字符串") "【平行样测试】" ("字符串") "【加标回收】" ("字符串") "【空白校准】" ("字符串") "【标样校准】" ("字符串") "【单步调试】" ("字符串") "【简易步骤】" ("字符串")] -> w430
          frame 0, Default {
            n257 = Number To Decimal String(number=w449) -> (decimal integer string=w448:string)  [unwired: 1 in]
          }
          frame 1 {
          }
          frame 2 {
          }
          frame 3 {
          }
          frame 4 {
          }
          frame 5 {
          }
          frame 6 {
          }
          frame 7 {
          }
          frame 8 {
          }
          frame 9 {
          }
          frame 254 {
          }
          frame 255 {
          }
        }
        n258 = global read "VAR总磷总氮全局变量.vi" "状态告警区"() -> (w440:T6)
        n259 = Unbundle By Name(w440) -> ("F0"=w439:sgl, "F1"=w438:sgl, "F2"=w437:sgl, "F3"=w436:sgl, "id"=w435:u16, "flowid"=w434:u16, "量程"=w433:u16)
        n260 = Concatenate Strings(w430, "停止" ("字符串"), ">>" ("字符串")) -> (w447:string)
        n261 = Format Into String(format string="F0=%#f,F1=%#f,F2=%#f,F3=%#f,Flow=%d-%-d-%-d" ("格式字符串"), w439, w438, w437, w436, w435, w434, w433) -> (resulting string=w431:string)  [unwired: 2 in, 1 out]
        n262 = call "id参数转换.vi"("id"=w442) -> ("table输出"=w441:string)  [unwired: 9 in, 1 out]
        n263 = Get Date/Time In Seconds() -> (seconds since 1Jan1904=w445:timestamp)
        n264 = Bundle By Name(cluster=T15 {"时间标识"=timestamp(0 s since 1904-01-01), "设备"="", "日志信息"="", "流程参数"=""} ("data in"), "时间标识"=w445, "设备"=w441, "日志信息"=w447, "流程参数"=w431) -> (w444:T15)
        n265 = call "总磷总氮操作日志.vi"("data in"=w444) -> ()  [unwired: 11 in]
      }
    }
    n266 = case shown="真" w417 {
      frame False {
      }
      frame True {
        n267 = property on="多列列表框" class="MCListbox (严格)"() -> ("ItemNames"=w489:string[][], "Value"=w485:i32)  [unwired: 2 in, 2 out]
        n268 = Index Array(array=w489, index (row)=w485) -> (element=w488:string[])  [unwired: 1 in]
        n269 = Index Array(array=w488) -> (element=w487:string)  [unwired: 1 in]
        n270 = call "过滤筛选流程.vi"("字符串"=w487) -> ("匹配后偏移量"=w486:i32)  [unwired: 10 in]
        n271 = case shown="默认" w486 {
          tunnel: w487 -> [w491 _]
          tunnel: w485 -> [w490 _]
          frame Default {
            n272 = case shown="默认" w491 {
              selector: w491 -> [w497 w504]
              tunnel: [w497 w504] -> w493
              tunnel: [string[] [] ("数组") w499] -> w492
              tunnel: w490 -> [_ w503]
              frame "读数" {
              }
              frame Default {
                n273 = Equal?(x=w503, y=1) -> (x = y?=w501:bool)
                n274 = Select(t=string[] [], s=w501, f="数组") -> (s? t:f=w499:string[])
              }
            }
            n275 = for {
              N: 1 -> [_]
              tunnel: w493 -> [w506]
              shift-right: [w505] -> w494
              shift-left: w492 -> [w507]
              n276 = Search 1D Array(1D array=w507, element=w506) -> (index of element=w510:i32)  [unwired: 1 in]
              n277 = Format Into String(format string="%s" ("格式字符串"), w506) -> (resulting string=w511:string)  [unwired: 2 in, 1 out]
              n278 = Equal?(x=w510, y=-1) -> (x = y?=w508:bool)
              n279 = case shown="真" w508 {
                tunnel: w511 -> [_ w521]
                tunnel: w507 -> [w513 w525]
                tunnel: w506 -> [_ w524]
                tunnel: [w513 w523] -> w505
                frame False {
                }
                frame True {
                  n280 = case shown="\"结束\"" w521 {
                    selector: w521 -> [w555 w558 w561]
                    tunnel: [w555 w557 w560] -> w520
                    frame Default {
                    }
                    frame "初始化" {
                      n281 = Concatenate Strings("<<--" ("字符串"), w558) -> (w557:string)
                    }
                    frame "结束" {
                      n282 = Concatenate Strings("-->>" ("字符串"), w561) -> (w560:string)
                    }
                  }
                  n283 = Insert Into Array(array=w525, new element=w524) -> (w523:string[])  [unwired: 1 in]
                  n284 = global read "VAR总磷总氮全局变量.vi" "状态告警区"() -> (w519:T6)
                  n285 = Unbundle By Name(w519) -> ("工作状态"=w518:u16)
                  n286 = case shown="0, 默认" w518 {
                    selector: w518 -> [w540 _ _ _ _ _ _ _ _ _ _ _]
                    tunnel: [w539 "【水样测试】" ("字符串") "【标样核查】" ("字符串") "【零点核查】" ("字符串") "【跨度核查】" ("字符串") "【空白测试】" ("字符串") "【平行样测试】" ("字符串") "【加标回收】" ("字符串") "【空白校准】" ("字符串") "【标样校准】" ("字符串") "【单步调试】" ("字符串") w551] -> w516
                    frame 0, Default {
                      n287 = Number To Decimal String(number=w540) -> (decimal integer string=w539:string)  [unwired: 1 in]
                    }
                    frame 1 {
                    }
                    frame 2 {
                    }
                    frame 3 {
                    }
                    frame 4 {
                    }
                    frame 5 {
                    }
                    frame 6 {
                    }
                    frame 7 {
                    }
                    frame 8 {
                    }
                    frame 9 {
                    }
                    frame 254 {
                    }
                    frame 255 {
                      n288 = local read "简易步骤名称"() -> (w553:string)
                      n289 = Format Into String(format string="(%s)" ("格式字符串"), initial string="【简易流程】" ("工作状态"), w553) -> (resulting string=w551:string)  [unwired: 1 in, 1 out]
                    }
                  }
                  n290 = global read "VAR总磷总氮全局变量.vi" "状态告警区"() -> (w538:T6)
                  n291 = global read "VAR总磷总氮全局变量.vi" "状态告警区"() -> (w535:T6)
                  n292 = Unbundle By Name(w535) -> ("F0"=w532:sgl, "F1"=w531:sgl, "F2"=w530:sgl, "F3"=w529:sgl, "id"=w528:u16, "flowid"=w527:u16, "量程"=w526:u16)
                  n293 = Unbundle By Name(w538) -> ("id"=w515:u16)
                  n294 = call "id参数转换.vi"("id"=w515) -> ("table输出"=w514:string)  [unwired: 9 in, 1 out]
                  n295 = Concatenate Strings(w516, w520) -> (w517:string)
                  n296 = Format Into String(format string="F0=%#f,F1=%#f,F2=%#f,F3=%#f,Flow=%d-%-d-%-d" ("格式字符串"), w532, w531, w530, w529, w528, w527, w526) -> (resulting string=w533:string)  [unwired: 2 in, 1 out]
                  n297 = Get Date/Time In Seconds() -> (seconds since 1Jan1904=w536:timestamp)
                  n298 = Bundle By Name(cluster=T15 {"时间标识"=timestamp(0 s since 1904-01-01), "设备"="", "日志信息"="", "流程参数"=""} ("data in"), "时间标识"=w536, "设备"=w514, "日志信息"=w517, "流程参数"=w533) -> (w537:T15)
                  n299 = call "总磷总氮操作日志.vi"("data in"=w537) -> ()  [unwired: 11 in]
                }
              }
            }
            n300 = local write "数组"(w494) -> ()
          }
          frame -1 {
          }
        }
      }
    }
    n301 = while {
      tunnel: w398 -> [w576]
      shift-right: [w571] -> _
      shift-left: _ -> [w573]
      shift-right: [w572] -> _
      shift-left: _ -> [w574]
      shift-right: [w562] -> _
      shift-left: _ -> [w570]
      tunnel: w399 -> [w564]
      shift-right: [w568] -> _
      shift-left: _ -> [w567]
      tunnel: w394 -> [w568]
      stop <- TRUE stop-if-true
      n302 = global read "总磷总氮断电保存全局变量.vi" "流程路径"() -> (w562:path)
      n303 = Not Equal?(x=w567, y=w568) -> (x != y?=w566:bool)
      n304 = Not Equal?(x=w570, y=w562) -> (x != y?=w565:bool)
      n305 = Not Equal To 0?(x=w564) -> (x != 0?=w563:bool)
      n306 = Compound Arithmetic op=OR ("复合运算")(w563, w565, w566) -> (w569:bool)
      n307 = case shown="真" w569 {
        tunnel: [w578 w588] -> w572
        tunnel: [w577 w587] -> w571
        tunnel: w576 -> [_ w582]
        tunnel: w574 -> [w578 _]
        tunnel: w573 -> [w577 _]
        tunnel: w562 -> [_ w581]
        tunnel: w564 -> [_ w580]
        frame False {
        }
        frame True {
          n308 = call "斯坦道XML解析.vi"("工作状态"=w580, "添加的路径"=w581, "参数簇"=w582) -> ("简易步骤名称"=→"简易步骤名称":string, "步骤时间"=w583:string[], "步骤名"=w585:string[])  [unwired: 6 in]
          n309 = for {
            tunnel: w585 -> [_] mode=indexing
            tunnel: [w589] -> w586 mode=indexing
            i -> [w589]
          }
          n310 = Build Array(w585, w583) -> (w584:string[][])
          n311 = Transpose 2D Array(2D array=w584) -> (transposed array=w587:string[][])
          n312 = Number To Decimal String(number=w586) -> (decimal integer string=w588:string[])  [unwired: 1 in]
        }
      }
      n313 = property on="多列列表框" class="MCListbox (严格)"("ItemNames"=w571, "RowHdrs[]"=w572) -> ()  [unwired: 2 in, 2 out]
    }
  }
  n314 = control-ref of="本VI"() -> (w9:refnum<vi>)
  n315 = property class="VI"(reference=w9) -> ("Library"=w10:refnum<vi>)  [unwired: 1 in, 2 out]
  n316 = property class="Library"(reference=w10) -> ("LocalName"=w7:string)  [unwired: 1 in, 2 out]
  n317 = while {
    stop <- FALSE stop-if-true
    n318 = control-ref of="试剂余量显示"() -> (w602:refnum<vi>)
    n319 = Wait (ms)(milliseconds to wait=u32 10000 ("等待时间（毫秒）")) -> ()  [unwired: 1 out]
    n320 = call "试剂余量展示.vi"("波形图 2"=w602) -> ("波形图"=→"试剂余量显示":sgl[][])  [unwired: 10 in]
  }
  n321 = Search/Split String(string=w7, search string/char (-)="." ("搜索字符串/字符(-)")) -> (substring before match=w5:string)  [unwired: 1 in, 2 out]
  n322 = call <vilib>:"Application Directory.vi"() -> ("Application Directory"=w11:path)
  n323 = Concatenate Strings(w5, "-" ("字符串"), "calibration.xml" ("名称或相对路径")) -> (w2:string)
  n324 = Build Path(base path=w11, name or relative path="data" ("名称或相对路径")) -> (appended path=w8:path)
  n325 = Build Path(base path=w8, name or relative path=w2) -> (appended path=w1:path)
  n326 = while {
    shift-right: [w607] -> _
    shift-left: _ -> [w609]
    tunnel: w1 -> [w606]
    stop <- FALSE stop-if-true
    n327 = Read from Text File(file (use dialog)=w606) -> (text=w607:string)  [unwired: 3 in, 3 out]
    n328 = Not Equal?(x=w609, y=w607) -> (x != y?=w608:bool)
    n329 = Wait (ms)(milliseconds to wait=u32 1000 ("等待时间（毫秒）")) -> ()  [unwired: 1 out]
    n330 = case shown="真" w608 {
      tunnel: w606 -> [_ _]
      frame False {
      }
      frame True {
        n331 = call "读取校准数据.vi"() -> ()  [unwired: 11 in, 1 out]
      }
    }
  }
  n332 = call "试剂余量后台任务.vi"() -> ()  [unwired: 12 in]
  n333 = Obtain Notifier(name (unnamed)=w18, notification data type=FALSE) -> (notifier out=w19:refnum<notifier>)  [unwired: 2 in, 2 out]
  n334 = Obtain Queue(name (unnamed)=w18, element data type=cluster{"命令":string, "data":variant} {"命令"="", "data"=variant}) -> (queue out=w23:refnum<queue>)  [unwired: 3 in, 2 out]
  n335 = while {
    tunnel: w23 -> [w619]
    stop <- FALSE stop-if-true
    n336 = Wait (ms)(milliseconds to wait=u32 1000 ("等待时间（毫秒）")) -> ()  [unwired: 1 out]
    n337 = global read "总磷总氮断电保存全局变量.vi" "MB通信方式选择"() -> (w617:enum16{"串口", "TCP"})
    n338 = global read "VAR总磷总氮全局变量.vi" "MB session in"() -> (w615:refnum<class "MB_Master.lvclass">)
    n339 = Get Queue Status(queue=w619) -> (queue out=w618:refnum<queue>, # elements in queue=w614:i32)  [unwired: 2 in, 6 out]
    n340 = case shown="\"串口\", 默认" w617 {
      tunnel: [w622 w623] -> w616
      frame "串口", Default {
        n341 = global read "总磷总氮断电保存全局变量.vi" "VISA Resource"() -> (w622:refnum<visa-resource-name>)
      }
      frame "TCP" {
        n342 = global read "总磷总氮断电保存全局变量.vi" "IP"() -> (w623:string)
      }
    }
    "字符串 2" <- w616
    n343 = property class="MB_Master"(reference=w615) -> ("Properties:Session Valid"=w613:bool)  [unwired: 1 in, 2 out]
    n344 = Equal To 0?(x=w614) -> (x = 0?=w612:bool)
    n345 = And(x=w612, y=w613) -> (x .and. y?=w611:bool)
    n346 = case shown="真" w611 {
      tunnel: w618 -> [_ w635]
      frame False {
      }
      frame True {
        n347 = global read "总磷总氮断电保存全局变量.vi" "启动队列名称"() -> (w624:cluster{"String":string, "Value":u16}[])
        n348 = for {
          tunnel: [w653] -> w625 mode=indexing
          tunnel: w624 -> [w654] mode=indexing
          n349 = Unbundle By Name(w654) -> ("Value"=w653:u16)
        }
        n350 = global read "VAR总磷总氮全局变量.vi" "状态告警区"() -> (w627:T6)
        n351 = Unbundle By Name(w627) -> ("系统时间"=w634:timestamp, "工作状态"=w626:u16)
        n352 = Get Date/Time In Seconds() -> (seconds since 1Jan1904=w633:timestamp)
        n353 = for {
          tunnel: w626 -> [w639]
          shift-right: [w640] -> w628
          shift-left: w635 -> [w642]
          tunnel: w625 -> [w636] mode=indexing
          n354 = Equal?(x=w639, y=T17."空闲") -> (x = y?=w637:bool)
          n355 = Bundle By Name(cluster=cluster{"命令":string, "data":variant} {"命令"="", "data"=variant} ("元素"), "命令"="读状态告警区", "data"=w636) -> (w644:cluster{"命令":string, "data":variant})
          n356 = Enqueue Element(queue=w642, element=w644) -> (queue out=w641:refnum<queue>)  [unwired: 2 in, 2 out]
          n357 = case shown="真" w637 {
            tunnel: w641 -> [w646 w649]
            tunnel: w636 -> [_ w648]
            tunnel: [w646 w647] -> w640
            frame False {
            }
            frame True {
              n358 = Bundle By Name(cluster=cluster{"命令":string, "data":variant} {"命令"="", "data"=variant} ("元素"), "命令"="读测量数据区", "data"=w648) -> (w651:cluster{"命令":string, "data":variant})
              n359 = Enqueue Element(queue=w649, element=w651) -> (queue out=w647:refnum<queue>)  [unwired: 2 in, 2 out]
            }
          }
        }
        n360 = Subtract(x=w633, y=w634) -> (x-y=w632:dbl)
        n361 = Absolute Value(x=w632) -> (abs(x)=w631:dbl)
        n362 = Greater Or Equal?(x=w631, y=120.0) -> (x >= y?=w629:bool)
        n363 = case shown="真" w629 {
          tunnel: w628 -> [_ w662]
          tunnel: [w655 _] -> _
          frame False {
            n364 = global read "VAR总磷总氮全局变量.vi" "MB session in"() -> (w660:refnum<class "MB_Master.lvclass">)
            n365 = call "序列号读取.vi"("MB session in"=w660) -> ("error out"=w658:errorcluster, "序列号"=w659:string, "MB session out"=w657:refnum<class "MB_Master.lvclass">)  [unwired: 8 in]
            n366 = global write "VAR总磷总氮全局变量.vi" "序列号"(w659) -> ()
            n367 = call "总磷总氮版本号读取.vi"("Error in"=w658, "MB session in"=w657) -> ("error out"=w655:errorcluster, "固件版本号"=→"固件版本号":string)  [unwired: 7 in, 1 out]
          }
          frame True {
            n368 = call "总磷总氮启动命令.vi"("参数"=T18 {"站号"=3, "量程切换"=enum."AUTO", "控制命令"=enum."校时", "模式设置"=enum."待机", "测量间隔"=0}) -> ("启动命令"=w661:cluster{"命令":string, "data":variant})  [unwired: 10 in]
            n369 = Enqueue Element(queue=w662, element=w661) -> ()  [unwired: 2 in, 3 out]
          }
        }
      }
    }
  }
  n370 = while {
    tunnel: w23 -> [w665]
    tunnel: w19 -> [w664]
    stop <- FALSE stop-if-true
    n371 = event shown="[5] \"布尔\": 鼠标按下" {
      selector: _ -> [_ _ _ _ _ _ _ _ _ _ _ _ _]
      dyn-events: _ -> [_ _ _ _ _ _ _ _ _ _ _ _ _]
      timeout: _ -> [_ _ _ _ _ _ _ _ _ _ _ _ _]
      tunnel: w665 -> [_ _ _ _ _ _ _ w673 _ w682 _ _ _]
      tunnel: w664 -> [_ _ _ _ _ _ _ _ _ w678 _ _ _]
      event Timeout {
        n372 = event-data() -> ()  [unwired: 1 in, 3 out]
      }
      event "温度曲线": Value Change {
        n373 = event-data() -> ()  [unwired: 1 in, 6 out]
        n374 = call "温度曲线显示.vi"() -> ()  [unwired: 12 in]
      }
      event "试剂余量": Value Change {
        n375 = event-data() -> ()  [unwired: 1 in, 6 out]
        n376 = call "试剂余量显示UI.vi"() -> ()  [unwired: 12 in]
      }
      event "灯值调整": Value Change {
        n377 = event-data() -> ()  [unwired: 1 in, 6 out]
        n378 = call "灯值调整对话框.vi"() -> ()  [unwired: 12 in]
      }
      event "启动参数设置": Value Change {
        n379 = event-data() -> ()  [unwired: 1 in, 6 out]
        n380 = call "启动参数设置.vi"() -> ()  [unwired: 12 in]
      }
      event "布尔": Mouse Down {
        n381 = event-data() -> ("CtlRef"=w668:refnum<vi>)  [unwired: 1 in, 5 out]
        n382 = property class="Bool (严格)"(reference=w668) -> ("Value"=w667:bool)  [unwired: 1 in, 2 out]
        n383 = case shown="假" w667 {
          frame False {
            n384 = call "密码键盘.vi"() -> ("NewNumber"=w669:u32)  [unwired: 1 in]
            n385 = global write "VAR总磷总氮全局变量.vi" "权限密码"(w669) -> ()
          }
          frame True {
            n386 = global write "VAR总磷总氮全局变量.vi" "权限密码"(u32 0 ("输入密码")) -> ()
          }
        }
      }
      event "流程固件": Value Change {
        n387 = event-data() -> ()  [unwired: 1 in, 6 out]
        n388 = call "流程固件设置对话框.vi"() -> ()  [unwired: 12 in]
      }
      event "手动启动": Value Change {
        n389 = event-data() -> ()  [unwired: 1 in, 6 out]
        n390 = call "总磷总氮启动参数对话框.vi"() -> ("确认"=w671:bool, "元素"=w672:cluster{"命令":string, "data":variant})  [unwired: 10 in]
        n391 = case shown="真" w671 {
          tunnel: w673 -> [_ w676]
          tunnel: w672 -> [_ w675]
          frame False {
          }
          frame True {
            n392 = Flush Queue(queue=w676) -> (queue out=w674:refnum<queue>)  [unwired: 1 in, 2 out]
            n393 = Enqueue Element(queue=w674, element=w675) -> ()  [unwired: 2 in, 3 out]
          }
        }
      }
      event "调试": Value Change {
        n394 = event-data() -> ()  [unwired: 1 in, 6 out]
        n395 = call "简易流程调试界面.vi"() -> ()  [unwired: 12 in]
      }
      event "停止": Value Change {
        n396 = event-data() -> ()  [unwired: 1 in, 6 out]
        n397 = Send Notification(notification=TRUE ("通知"), notifier=w678) -> ()  [unwired: 1 in, 2 out]
        n398 = Enqueue Element(queue=w682, element=cluster{"命令":string, "data":variant} {"命令"="启动", "data"=variant(cluster{"站号":u16, "控制命令输出":u16[]} {"站号"=1, "控制命令输出"=[2816]})} ("元素")) -> (queue out=w679:refnum<queue>)  [unwired: 2 in, 2 out]
        n399 = Enqueue Element(queue=w679, element=cluster{"命令":string, "data":variant} {"命令"="启动", "data"=variant(cluster{"站号":u16, "控制命令输出":u16[]} {"站号"=2, "控制命令输出"=[2816]})} ("元素")) -> ()  [unwired: 2 in, 3 out]
      }
      event "参数设置", "参数查询": Value Change {
        n400 = event-data() -> ()  [unwired: 1 in, 6 out]
        n401 = vi-ref "参数设置页.vi"() -> (w684:refnum<vi>)
        n402 = property on="窗格" class="Pane"("Origin"=T9 {"Horizontal"=0, "Vertical"=640} ("原点")) -> ()  [unwired: 2 in, 2 out]
        n403 = property class="VI"(reference=w684) -> (reference out=w686:refnum<vi>, "Exec.State"=w685:T7)  [unwired: 1 in, 1 out]
        n404 = case shown="\"Bad\", 默认" w685 {
          tunnel: w686 -> [w689 w693]
          tunnel: [w689 w690] -> w687
          frame "Bad", Default {
          }
          frame "Idle" {
            n405 = invoke class="VI" method="Run VI"(reference=w693, "Wait until done"=FALSE ("结束前等待"), "Auto Dispose Ref"=TRUE ("自动销毁引用")) -> (reference out=w690:refnum<vi>)  [unwired: 2 in, 4 out]
          }
        }
        n406 = invoke on="子面板" class="SubPnl" method="Remove VI"() -> (error out=w683:errorcluster)  [unwired: 3 in, 2 out]
        n407 = invoke on="子面板" class="SubPnl" method="Insert VI"(error in=w683, "VI Ref"=w687) -> ()  [unwired: 2 in, 4 out]
      }
      event "仪器校准": Value Change {
        n408 = event-data() -> ()  [unwired: 1 in, 6 out]
        n409 = vi-ref "校准设置页.vi"() -> (w695:refnum<vi>)
        n410 = property class="VI"(reference=w695) -> (reference out=w697:refnum<vi>, "Exec.State"=w696:T7)  [unwired: 1 in, 1 out]
        n411 = case shown="\"Bad\", 默认" w696 {
          tunnel: w697 -> [w699 w703]
          tunnel: [w699 w700] -> w698
          frame "Bad", Default {
          }
          frame "Idle" {
            n412 = invoke class="VI" method="Run VI"(reference=w703, "Wait until done"=FALSE ("结束前等待"), "Auto Dispose Ref"=TRUE ("自动销毁引用")) -> (reference out=w700:refnum<vi>)  [unwired: 2 in, 4 out]
          }
        }
        n413 = invoke on="子面板" class="SubPnl" method="Remove VI"() -> (error out=w694:errorcluster)  [unwired: 3 in, 2 out]
        n414 = invoke on="子面板" class="SubPnl" method="Insert VI"(error in=w694, "VI Ref"=w698) -> ()  [unwired: 2 in, 4 out]
      }
      event "返回": Value Change {
        n415 = event-data() -> ()  [unwired: 1 in, 6 out]
        n416 = property on="窗格" class="Pane"("Origin"=T9 {"Horizontal"=0, "Vertical"=0} ("原点")) -> ()  [unwired: 2 in, 2 out]
      }
    }
  }
